vi "Shoot.vi"(1 "Current Motor SetPoint":dbl=-0.5789538215358933, 2 "Current Angle":dbl=88.59692143572622) -> (0 "New Motor Setpoint":dbl)   [LabVIEW 2013]
uses:
  Robot Global Data.vi
panel:
  in  "Launch Parameters":dbl[][](array[numeric])=[[0.1, 1.0, 1.0, 1.0, 1.0], [170.0, 130.0, 135.0, 140.0, 135.0]]
  in  "Coast Bias":dbl=0.3 format="%#_13g"
  out "Cycle time":u32=827
  out "Shoot time":u32=552
  out "Meas. Angle":cluster{"Angle":dbl, dbl}(graph)={"Angle"=162.8219498163606, 170.1646174357262}
  out "Encoder Rate (deg/sec)":dbl=203.93229166666663
  out "Meas. Speed":T1(graph)
  out "Error":dbl=0.5
  in  "Speed Gain":dbl=0.003 step=0.0005
  in  "Measured Rate":dbl
  in  "Desired Rate":dbl=50.0
  # "Speeds"
  # "Angles"
  # "A   \nLow Goal"
  # "B   \nTruss"
  # "X\nHigh Goal 1"
  # "Y\nHigh Goal 2"
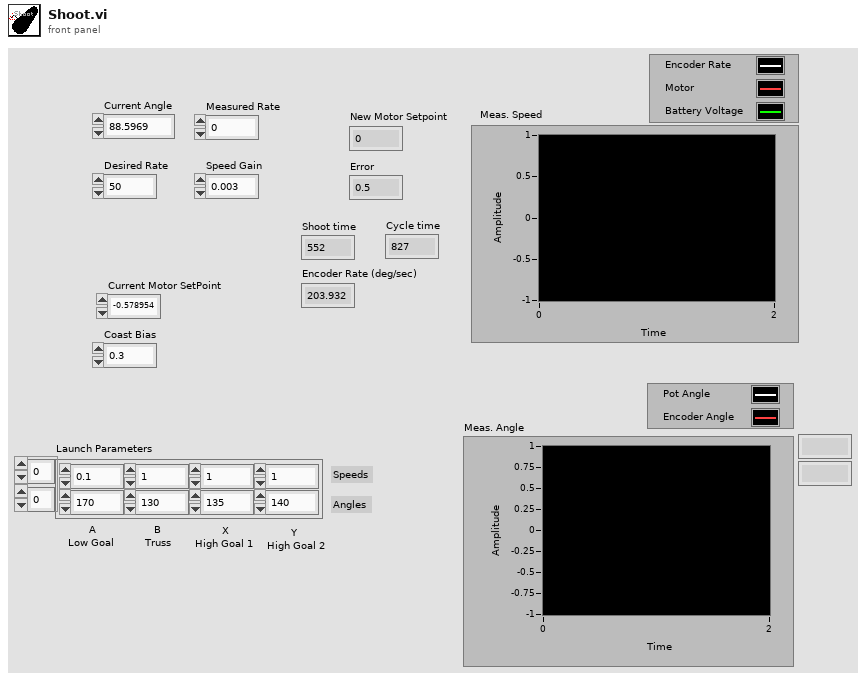
[diagram p1: front panel]
types:
  T1 = cluster{"Rate":dbl, dbl, "robot battery voltage":dbl}
  T2 = typedef "WPI_EncoderDevRef.ctl" = cluster{"DevStatus":errorcluster, "EncoderIndex":T3, "CounterIndex":T4, "DistancePerCount":dbl, "Decoding Type":T5}
  T3 = typedef "FPGA_EncoderIdx.ctl" = enum8{"Enc 0", "Enc 1", "Enc 2", "Enc 3", "Invalid"}
  T4 = typedef "FPGA_CounterCtrSystemIndex.ctl" = enum8{"Ctr 0", "Ctr 1", "Ctr 2", "Ctr 3", "Ctr 4", "Ctr 5", "Ctr 6", "Ctr 7", "Invalid"}
  T5 = typedef "WPI_EncoderType.ctl" = enum16{"1x", "2x", "4x"}
  T6 = enum16{"Hold", "Pick Up", "Catch", "Aim", "Shoot", "Joystick"}
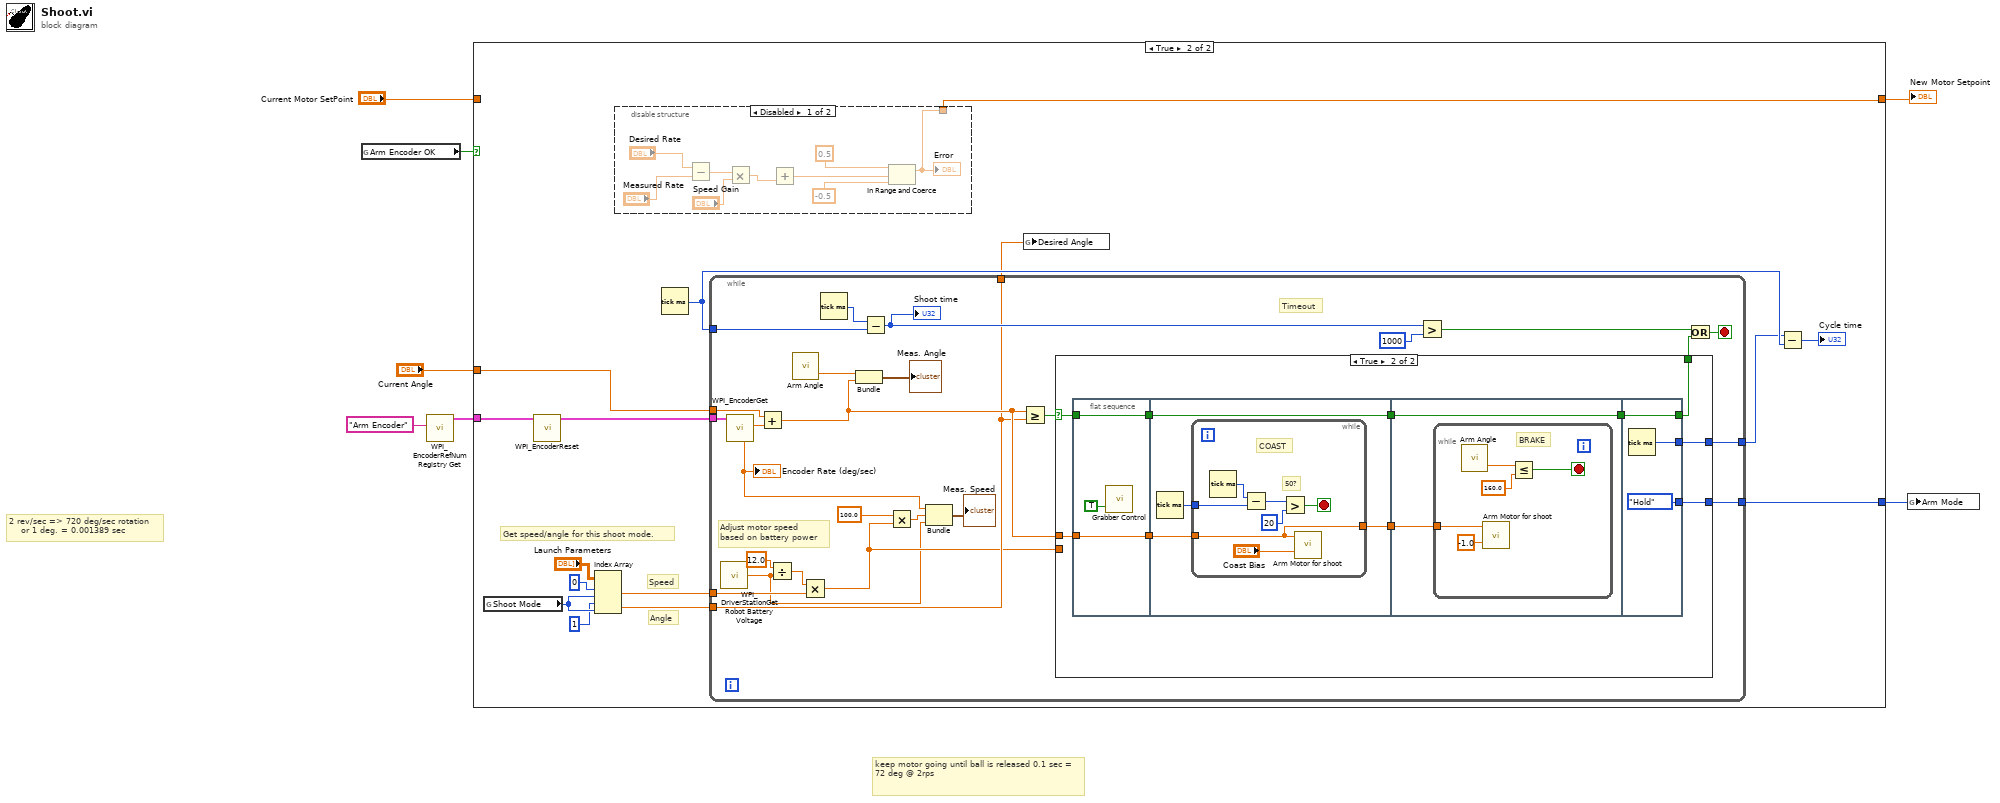
[diagram p0: block diagram]
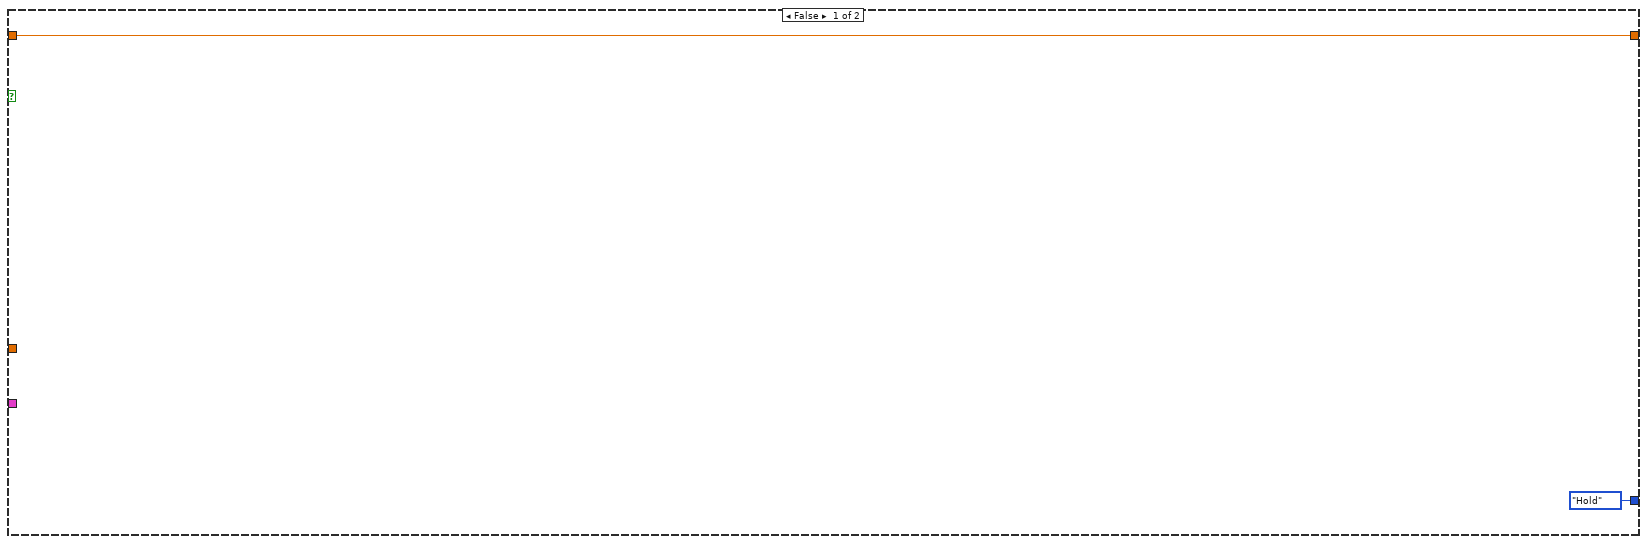
[diagram p2: hidden frame]
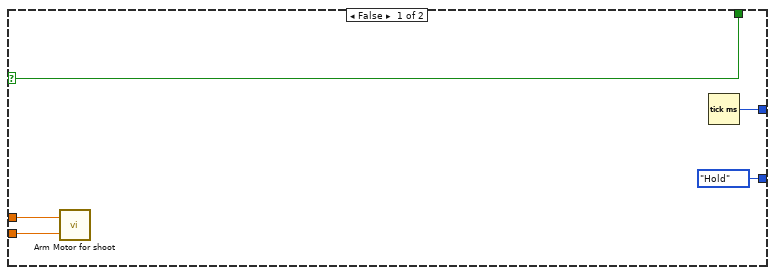
[diagram p4: hidden frame]
diagram:
  # "keep motor going until ball is released 0.1 sec = 72 deg @ 2rps"
  # "2 rev/sec => 720 deg/sec rotation\n    or 1 deg. = 0.001389 sec"
  n1 = global read "Robot Global Data.vi" "Arm Encoder OK"() -> (w2:bool)
  n2 = call <vilib>:"WPI_EncoderRefNum Registry Get.vi"("refnum name"="Arm Encoder") -> ("EncoderDevRef"=w3:T2)  [unwired: 9 in, 1 out]
  n3 = case shown="True" w2 {
    tunnel: "Current Motor SetPoint" -> [w9 _]
    tunnel: [w9 w21] -> w6
    tunnel: w3 -> [_ w20]
    tunnel: "Current Angle" -> [_ w18]
    tunnel: [T6."Hold" ("Arm Mode") w10] -> w1
    frame False {
    }
    frame True {
      # "Angle"
      # "Speed"
      # "Get speed/angle for this shoot mode."
      n4 = global read "Robot Global Data.vi" "Shoot Mode"() -> (w16:i8)
      n5 = call <vilib>:"WPI_EncoderReset.vi"("EncoderDevRef"=w20) -> ("EncoderDevRef"=w19:T2)  [unwired: 9 in, 1 out]
      n6 = Index Array(array="Launch Parameters", index (row) #1=0 ("disabled index (row)"), index (col) #1=w16, index (row) #2=1 ("disabled index (row)"), index (col) #2=w16) -> (element #1=w13:dbl, element #2=w12:dbl)
      n7 = disable-structure shown="Disabled" {
        disable-tunnel: [w28 _] -> w21
        frame Disabled {
          n8 = Subtract(x="Desired Rate", y="Measured Rate") -> (x-y=w33:dbl)
          n9 = Multiply(x=w33, y="Speed Gain") -> (x*y=w26:dbl)
          n10 = Add(y=w26) -> (x+y=w27:dbl)  [unwired: 1 in]
          n11 = In Range and Coerce(upper limit=0.5, x=w27, lower limit=-0.5) -> (coerced(x)=w28:dbl)  [unwired: 1 out]
          "Error" <- w28
        }
        frame Enabled {
        }
      }
      n12 = Tick Count (ms)() -> (millisecond timer value=w24:u32)
      n13 = while {
        tunnel: w24 -> [w56]
        tunnel: w19 -> [w55]
        tunnel: [w45] -> w22
        tunnel: w18 -> [w51]
        tunnel: w13 -> [w37]
        tunnel: w12 -> [w41]
        tunnel: [w41] -> w11
        tunnel: [w40] -> w10
        stop <- w52 stop-if-true
        # "Adjust motor speed\nbased on battery power"
        # "Timeout"
        n14 = call <vilib>:"WPI_DriverStationGet Robot Battery Voltage.vi"() -> ("robot battery voltage"=w35:dbl)  [unwired: 14 in, 1 out]
        n15 = call <vilib>:"WPI_EncoderGet.vi"("EncoderDevRef"=w55) -> ("Distance"=w54:dbl, "Rate"=w39:dbl)  [unwired: 1 in, 8 out]
        "Encoder Rate (deg/sec)" <- w39
        n16 = Add(x=w51, y=w54) -> (x+y=w42:dbl)
        n17 = Divide(x=12.0, y=w35) -> (x/y=w36:dbl)
        n18 = call "Arm Angle.vi"() -> ("Angle"=w43:dbl)  [unwired: 2 in, 1 out]
        n19 = Multiply(x=w36, y=w37) -> (x*y=w38:dbl)
        n20 = Tick Count (ms)() -> (millisecond timer value=w57:u32)
        n21 = Bundle("Angle"=w43, w42) -> (→"Meas. Angle":cluster{"Angle":dbl, dbl})  [unwired: 1 in]
        n22 = Subtract(x=w57, y=w56) -> (x-y=w59:u32)
        "Shoot time" <- w59
        n23 = Multiply(x=100.0, y=w38) -> (x*y=w49:dbl)
        n24 = Bundle("Rate"=w39, w49, "robot battery voltage"=w35) -> (→"Meas. Speed":T1)  [unwired: 1 in]
        n25 = Greater Or Equal?(x=w42, y=w41) -> (x >= y?=w47:bool)
        n26 = case shown="True" w47 {
          selector: w47 -> [w62 w66]
          tunnel: w42 -> [w64 w74]
          tunnel: [w62 w70] -> w46
          tunnel: [w63 w73] -> w45
          tunnel: w38 -> [w61 _]
          tunnel: [T6."Hold" ("Arm Mode") w65] -> w40
          frame False {
            n27 = call "Arm Motor for shoot.vi"("Motor input"=w61, "Current angle (deg)"=w64) -> ()  [unwired: 1 in]
            n28 = Tick Count (ms)() -> (millisecond timer value=w63:u32)
          }
          frame True {
            n29 = flat-sequence {
              tunnel: w74 -> [w77]
              tunnel: [w77] -> w71
              tunnel: [w76] -> w67
              tunnel: w66 -> [w76]
              tunnel: [w79] -> w72
              tunnel: w71 -> [w80]
              tunnel: [w78] -> w68
              tunnel: w67 -> [w78]
              tunnel: w72 -> [w90]
              tunnel: [w89] -> w69
              tunnel: w68 -> [w89]
              tunnel: [w98] -> w73
              tunnel: [w97] -> w70
              tunnel: w69 -> [w97]
              tunnel: [T6."Hold" ("Arm Mode")] -> w65
              frame #0 {
                n30 = call "Grabber Control.vi"("Forcing"=TRUE ("Shooting")) -> ()  [unwired: 2 in]
              }
              frame #1 {
                n31 = Tick Count (ms)() -> (millisecond timer value=w81:u32)
                n32 = while {
                  tunnel: w80 -> [w82]
                  tunnel: w81 -> [w87]
                  tunnel: [w82] -> w79
                  stop <- w83 stop-if-true
                  # "COAST"
                  # "50?"
                  n33 = Tick Count (ms)() -> (millisecond timer value=w86:u32)
                  n34 = Subtract(x=w86, y=w87) -> (x-y=w85:u32)
                  n35 = Greater?(x=w85, y=u32 20 ("milliseconds to wait")) -> (0:w83:bool)
                  n36 = call "Arm Motor for shoot.vi"("Motor input"="Coast Bias", "Current angle (deg)"=w82) -> ()  [unwired: 1 in]
                }
              }
              frame #2 {
                n37 = while {
                  tunnel: w90 -> [w95]
                  stop <- w92 stop-if-true
                  # "BRAKE"
                  n38 = call "Arm Angle.vi"() -> ("Angle"=w93:dbl)  [unwired: 2 in, 1 out]
                  n39 = call "Arm Motor for shoot.vi"("Motor input"=-1.0, "Current angle (deg)"=w95) -> ()  [unwired: 1 in]
                  n40 = Less Or Equal?(x=w93, y=160.0) -> (x <= y?=w92:bool)
                }
              }
              frame #3 {
                n41 = Tick Count (ms)() -> (millisecond timer value=w98:u32)
              }
            }
          }
        }
        n42 = Greater?(x=w59, y=u32 1000) -> (0:w53:bool)
        n43 = Or(x=w53, y=w46) -> (x .or. y?=w52:bool)
      }
      n44 = global write "Robot Global Data.vi" "Desired Angle"(w11) -> ()
      n45 = Subtract(x=w22, y=w24) -> (x-y=→"Cycle time":u32)
    }
  }
  "New Motor Setpoint" <- w6
  n46 = global write "Robot Global Data.vi" "Arm Mode"(w1) -> ()
